vi "WSVCAP SHL Host TL RFFE Write - Single DUT.vi"(0 "Data Out":string, 11 "error in":errorcluster, 12 "Log (T)":bool=TRUE, 13 "DUT":T1) -> (15 "error out":errorcluster)   [LabVIEW 2012]
uses:
  Type Defs/WSVCAP SHL DUT Number Enum.ctl
panel:
  out "Socket Mask":u16=1 format="%02x"
  out "RFFE Data Out":u8[][](array[numeric]) format="%02x"
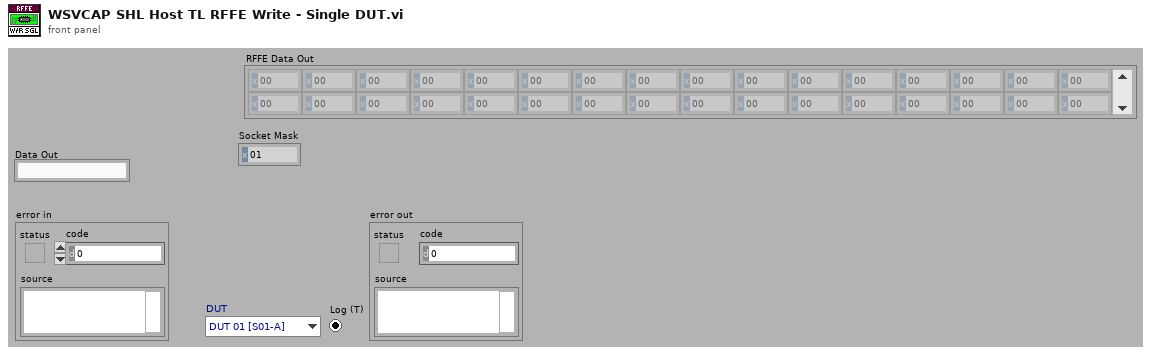
[diagram p1: front panel]
types:
  T1 = typedef "WSVCAP SHL DUT Number Enum.ctl" = enum16{"DUT 01 [S01-A]", "DUT 02 [S02-B]", "DUT 03 [S03-C]", "DUT 04 [S04-D]", "DUT 05 [S05-E]", "DUT 06 [S06-F]", "DUT 07 [S07-G]", "DUT 08 [S08-H]", "DUT 09 [S09-I]", "DUT 10 [S10-J]", "DUT 11 [S11-K]", "DUT 12 [S12-L]", "DUT 13 [S13-M]", "DUT 14 [S14-N]", "DUT 15 [S15-O]", "DUT 16 [S16-P]"}
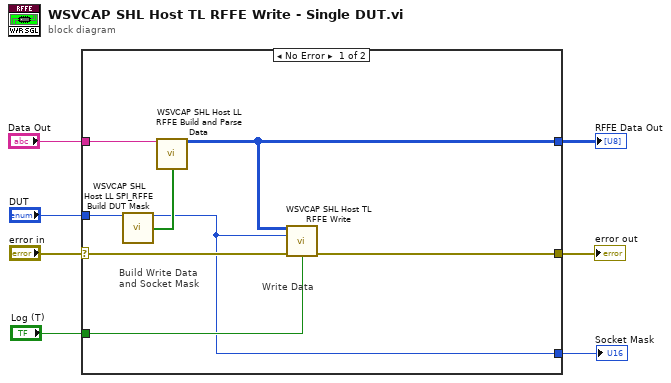
[diagram p0: block diagram]
diagram:
  n1 = case shown="No Error" "error in" {
    selector: "error in" -> [w14 _]
    tunnel: [w13 _] -> w7
    tunnel: "Data Out" -> [w12 _]
    tunnel: [w10 _] -> w4
    tunnel: "DUT" -> [w15 _]
    tunnel: [w8 _] -> w2
    tunnel: "Log (T)" -> [w9 _]
    frame No Error {
      # "Write Data"
      # "Build Write Data and Socket Mask"
      n2 = call "WSVCAP SHL Host LL SPI_RFFE Build DUT Mask.vi"("DUT"=w15) -> ("Socket Mask [U16]"=w8:u16, "DUT Mask"=w11:bool[])  [unwired: 12 in, 1 out]
      n3 = call "WSVCAP SHL Host LL RFFE Build and Parse Data.vi"("Data Out"=w12, "DUT Mask (All)"=w11) -> ("RFFE Data Out [U8]"=w10:u8[][])  [unwired: 10 in, 3 out]
      n4 = call "WSVCAP SHL Host TL RFFE Write.vi"("RFFE Data Out"=w10, "Socket Mask"=w8, "error in"=w14, "Log (T)"=w9) -> ("error out"=w13:errorcluster)  [unwired: 11 in]
    }
    frame Error {
    }
  }
  "error out" <- w7
  "RFFE Data Out" <- w4
  "Socket Mask" <- w2
